vi "cam_fgv.vi"(7 "cmd":enum16{"ini", "grab", "close"}(ring), 8 "error in":errorcluster, 11 "Image In":T2) -> (0 "error out":errorcluster, 3 "Image Out":T2)   [LabVIEW 2016]
uses:
  <vilib>/vision/Image Controls.llb/IMAQ Image.ctl
  <vilib>/userdefined/High Color/IMAQdx.ctl
  <vilib>/vision/driver/NI_Vision_Acquisition_Software.lvlib
  <resource>/objmgr/imaqdx.rc
panel:
  in  "Session In":T1="FDC"
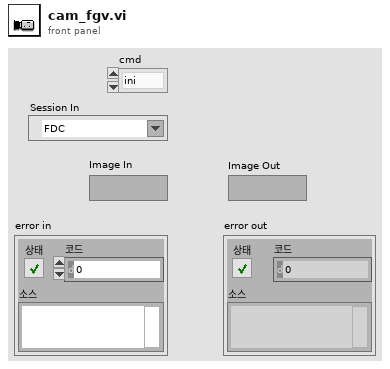
[diagram p1: front panel]
types:
  T1 = typedef "IMAQdx.ctl" = refnum<k21>
  T2 = typedef "IMAQ Image.ctl" = refnum<image>
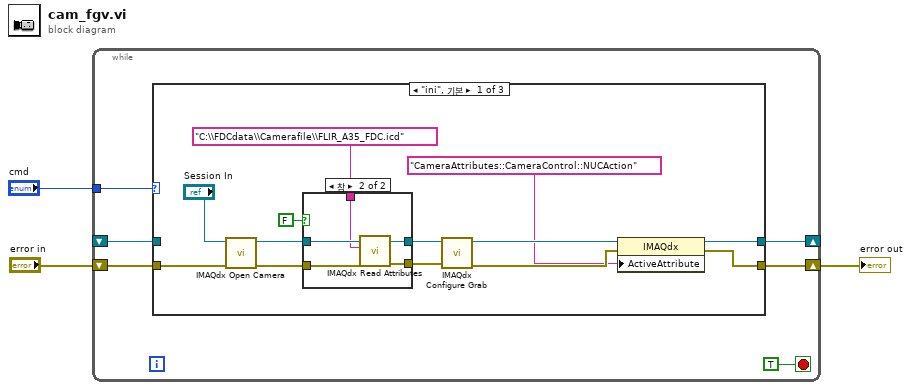
[diagram p0: block diagram]
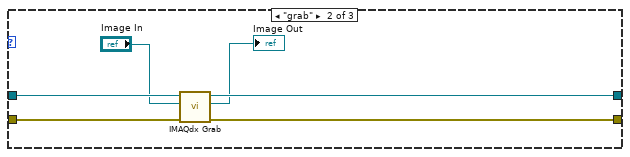
[diagram p3: hidden frame]
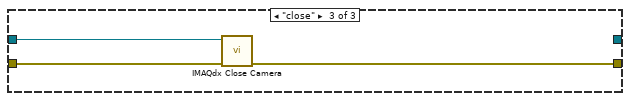
[diagram p4: hidden frame]
diagram:
  n1 = while {
    tunnel: "cmd" -> [w8]
    shift-right: [w6] -> w1
    shift-left: "error in" -> [w7]
    shift-right: [w5] -> _
    shift-left: _ -> [w4]
    stop <- TRUE stop-if-true
    n2 = case shown="\"ini\", 기본" w8 {
      tunnel: w7 -> [w21 w34 w37]
      tunnel: [w12 w33 w36] -> w6
      tunnel: [w11 w32 _] -> w5
      tunnel: w4 -> [_ w35 w38]
      frame "ini", Default {
        n3 = call <vilib>:"IMAQdx Open Camera.vi"("error in"=w21, "Session In"="Session In") -> ("error out"=w20:errorcluster, "Session Out"=w17:T1)  [unwired: 8 in]
        n4 = case shown="참" FALSE {
          tunnel: w20 -> [w23 w29]
          tunnel: [w23 w28] -> w19
          tunnel: [w24 w27] -> w18
          tunnel: w17 -> [w24 w26]
          tunnel: "C:\\FDCdata\\Camerafile\\FLIR_A35_FDC.icd" ("Filename") -> [_ w25]
          frame False {
          }
          frame True {
            n5 = call <vilib>:"IMAQdx Read Attributes.vi"("error in"=w29, "Filename"=w25, "Session In"=w26) -> ("error out"=w28:errorcluster, "Session Out"=w27:T1)  [unwired: 7 in]
          }
        }
        n6 = call <vilib>:"IMAQdx Configure Grab.vi"("error in"=w19, "Session In"=w18) -> ("error out"=w13:errorcluster, "Session Out"=w14:T1)  [unwired: 8 in]
        n7 = property class="IMAQdx"(reference=w14, error in=w13, "ActiveAttribute"="CameraAttributes::CameraControl::NUCAction") -> (reference out=w11:T1, error out=w12:errorcluster)
      }
      frame "grab" {
        n8 = call <vilib>:"IMAQdx Grab.vi"("error in"=w34, "Image In"="Image In", "Session In"=w35) -> ("error out"=w33:errorcluster, "Image Out"=→"Image Out":T2, "Session Out"=w32:T1)  [unwired: 5 in, 1 out]
      }
      frame "close" {
        n9 = call <vilib>:"IMAQdx Close Camera.vi"("error in"=w37, "Session In"=w38) -> ("error out"=w36:errorcluster)  [unwired: 9 in]
      }
    }
  }
  "error out" <- w1
